vi "Distance between points.vi"(2 "Position 2":cluster{"x":i32, "y":i32}, 3 "Position 1":cluster{"x":i32, "y":i32}) -> (0 "Distance":dbl)   [LabVIEW 2014, in "COSYLib.lvlib"]
uses:
  COSYLib.lvlib
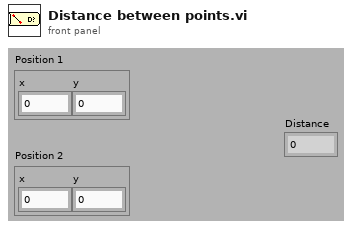
[diagram p1: front panel]
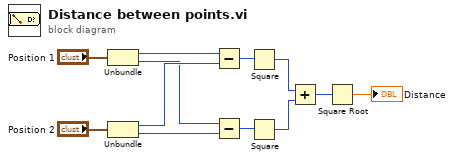
[diagram p0: block diagram]
diagram:
  n1 = Unbundle("Position 1") -> ("x"=w4:i32, "y"=w2:i32)
  n2 = Unbundle("Position 2") -> ("x"=w3:i32, "y"=w1:i32)
  n3 = Subtract(x=w4, y=w3) -> (x-y=w7:i32)
  n4 = Subtract(x=w2, y=w1) -> (x-y=w8:i32)
  n5 = Square(x=w7) -> (x^2=w9:i32)
  n6 = Square(x=w8) -> (x^2=w10:i32)
  n7 = Add(x=w9, y=w10) -> (x+y=w11:i32)
  n8 = Square Root(x=w11) -> (sqrt(x)=→"Distance":dbl)
